vi "GetPSUStatus.vi"(8 "error in (no error)":errorcluster, 11 "PSU_N87 in":refnum<class "PSU_N87.lvclass">) -> (0 "error out":errorcluster, 1 "OCP Tripped":bool, 2 "OVP Tripped":bool, 3 "PSU_N87 out":refnum<class "PSU_N87.lvclass">, 4 "Current (A)":dbl, 5 "Voltage (V)":dbl)   [LabVIEW 2014, in "PSU_N87.lvclass"]
uses:
  PSU_N87.lvclass
  PSU_N87.lvclass/PSU_N87.ctl
  <instrlib>/Agilent N87XX Series/Agilent N87XX Series.lvlib
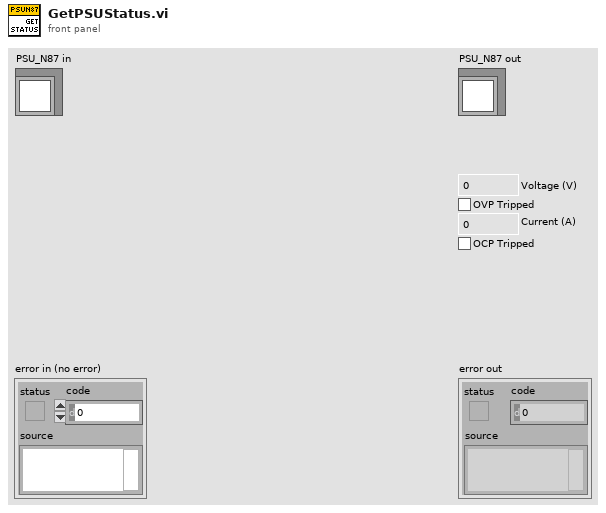
[diagram p1: front panel]
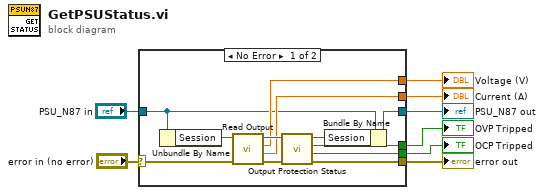
[diagram p0: block diagram]
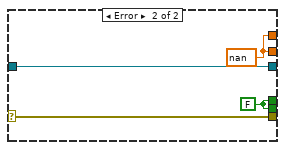
[diagram p2: hidden frame]
diagram:
  n1 = case shown="No Error" "error in (no error)" {
    selector: "error in (no error)" -> [w12 w24]
    tunnel: "PSU_N87 in" -> [w11 w23]
    tunnel: [w18 w22] -> w7
    tunnel: [w17 w22] -> w6
    tunnel: [w16 w21] -> w5
    tunnel: [w15 w21] -> w4
    tunnel: [w13 w24] -> w3
    tunnel: [w10 w23] -> w1
    frame No Error {
      n2 = Unbundle By Name(w11) -> ("Session"=w20:refnum<visa-resource-name>)
      n3 = call <instrlib>:"Read Output.vi"("error in (no error)"=w12, "VISA resource name"=w20) -> ("error out"=w14:errorcluster, "Actual Current Level (A)"=w17:dbl, "Actual Voltage Level (V)"=w18:dbl, "VISA resource name out"=w19:refnum<visa-resource-name>)  [unwired: 6 in]
      n4 = call <instrlib>:"Output Protection Status.vi"("error in (no error)"=w14, "VISA resource name"=w19) -> ("error out"=w13:errorcluster, "OCP Tripped?"=w15:bool, "OVP Tripped?"=w16:bool, "VISA resource name out"=w9:refnum<visa-resource-name>)  [unwired: 5 in, 1 out]
      n5 = Bundle By Name(cluster=w11, "Session"=w9) -> (w10:refnum<class "PSU_N87.lvclass">)
    }
    frame Error {
      w21 = FALSE ("OVP Tripped?")
      w22 = nan ("Actual Voltage Level (V)")
    }
  }
  "error out" <- w3
  "PSU_N87 out" <- w1
  "Voltage (V)" <- w7
  "Current (A)" <- w6
  "OCP Tripped" <- w4
  "OVP Tripped" <- w5
